vi "Update DVR API Contents.vi"(8 "error in (no error)":errorcluster, 9 "Class DVR Control File Path":path, 10 "Method Path":path, 11 "DVR API Path":path) -> (0 "error out":errorcluster, 3 "DVR VI Path":path)   [LabVIEW 2016, in "SLL Class DVR API Generator.lvlib"]
uses:
  SLL Class DVR API Generator.lvlib
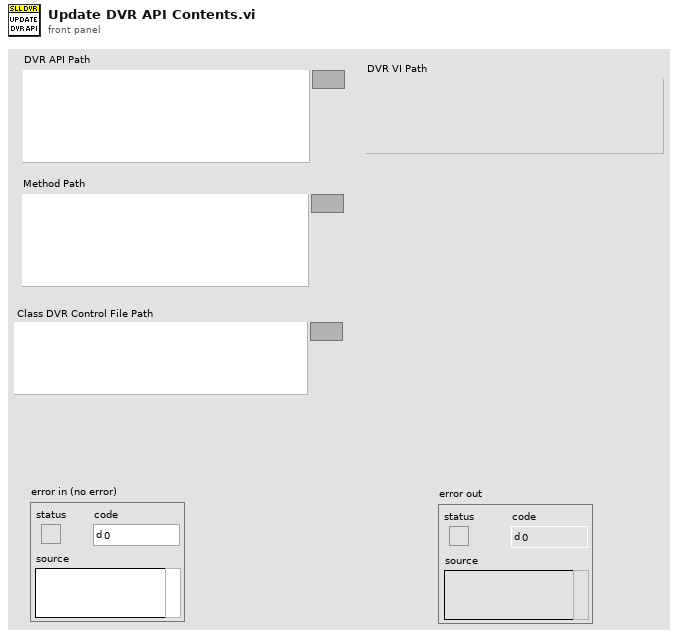
[diagram p1: front panel]
types:
  T1 = typedef "LVPositionTypeDef.ctl" = cluster{"Left":i32, "Top":i32}
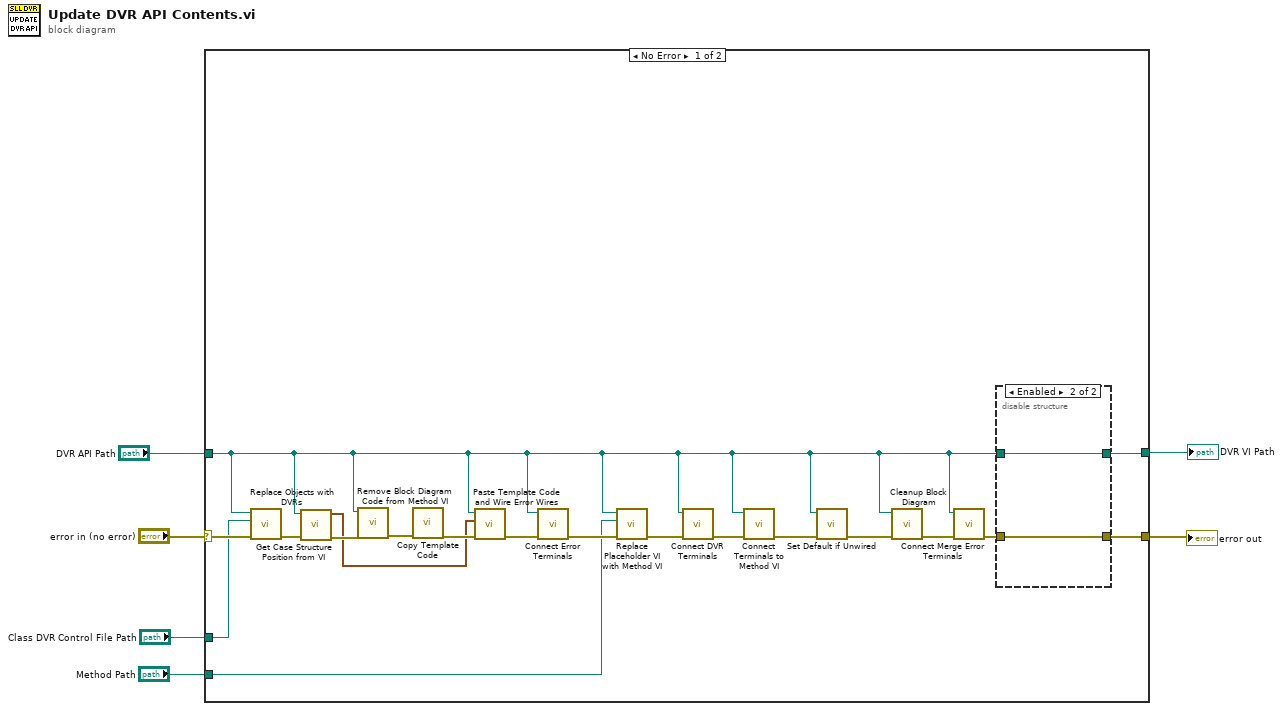
[diagram p0: block diagram]
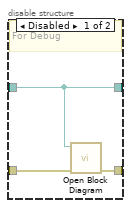
[diagram p2: hidden frame]
diagram:
  n1 = case shown="No Error" "error in (no error)" {
    selector: "error in (no error)" -> [w25 w32]
    tunnel: [w21 w32] -> w5
    tunnel: "DVR API Path" -> [w7 w31]
    tunnel: "Class DVR Control File Path" -> [w24 _]
    tunnel: "Method Path" -> [w18 _]
    tunnel: [w12 w31] -> w1
    frame No Error {
      n2 = call "Replace Objects with DVRs.vi"("error in (no error)"=w25, "Class DVR Control File Path"=w24, "DVR API Path"=w7) -> ("error out"=w11:errorcluster)  [unwired: 7 in, 1 out]
      n3 = call "Get Case Structure Position from VI.vi"("error in (no error)"=w11, "Method VI Path"=w7) -> ("error out"=w10:errorcluster, "Position"=w9:T1)  [unwired: 8 in]
      n4 = call "Remove Block Diagram Code from Method VI.vi"("error in (no error)"=w10, "Method VI Path"=w7) -> ("error out"=w23:errorcluster)  [unwired: 9 in]
      n5 = call "Copy Template Code.vi"("error in (no error)"=w23) -> ("error out"=w22:errorcluster)  [unwired: 10 in]
      n6 = call "Paste Template Code and Wire Error Wires.vi"("error in (no error)"=w22, "Position"=w9, "DVR API Path"=w7) -> ("error out"=w19:errorcluster)  [unwired: 8 in]
      n7 = call "Connect Error Terminals.vi"("error in (no error)"=w19, "VI Path"=w7) -> ("error out"=w20:errorcluster)  [unwired: 9 in]
      n8 = call "Replace Placeholder VI with Method VI.vi"("error in (no error)"=w20, "Method VI Path"=w18, "DVR VI Path"=w7) -> ("error out"=w17:errorcluster)  [unwired: 8 in]
      n9 = call "Connect DVR Terminals.vi"("error in (no error)"=w17, "DVR VI Path"=w7) -> ("error out"=w15:errorcluster)  [unwired: 9 in]
      n10 = call "Connect Terminals to Method VI.vi"("error in (no error)"=w15, "DVR VI Path"=w7) -> ("error out"=w16:errorcluster)  [unwired: 9 in]
      n11 = call "Set Default if Unwired.vi"("error in (no error)"=w16, "VI Path"=w7) -> ("error out"=w14:errorcluster)  [unwired: 9 in]
      n12 = call "Cleanup Block Diagram.vi"("error in (no error)"=w14, "VI Path"=w7) -> ("error out"=w13:errorcluster)  [unwired: 8 in, 1 out]
      n13 = call "Connect Merge Error Terminals.vi"("error in (no error)"=w13, "DVR VI Path"=w7) -> ("error out"=w8:errorcluster)  [unwired: 9 in]
      n14 = disable-structure shown="Enabled" {
        disable-tunnel: [w28 w30] -> w21
        disable-tunnel: w8 -> [w27 w30]
        disable-tunnel: w7 -> [w26 w29]
        disable-tunnel: [w26 w29] -> w12
        frame Disabled {
          # "For Debug"
          n15 = call "Open Block Diagram.vi"("error in (no error)"=w27, "VI Path"=w26) -> ("error out"=w28:errorcluster)  [unwired: 8 in, 1 out]
        }
        frame Enabled {
        }
      }
    }
    frame Error {
    }
  }
  "error out" <- w5
  "DVR VI Path" <- w1
